vi "Compile Script.vi"(0 "scripts manager in":refnum<class "scripts manager.lvclass">, 11 "error in (no error)":errorcluster) -> (4 "scripts manager out":refnum<class "scripts manager.lvclass">, 15 "error out":errorcluster)   [LabVIEW 2019, in "LSL.lvlib" / "scripts manager.lvclass"]
uses:
  scripts manager.lvclass
  scripts manager.lvclass/scripts manager.ctl
  output terminal/Base/Output Terminal.lvclass
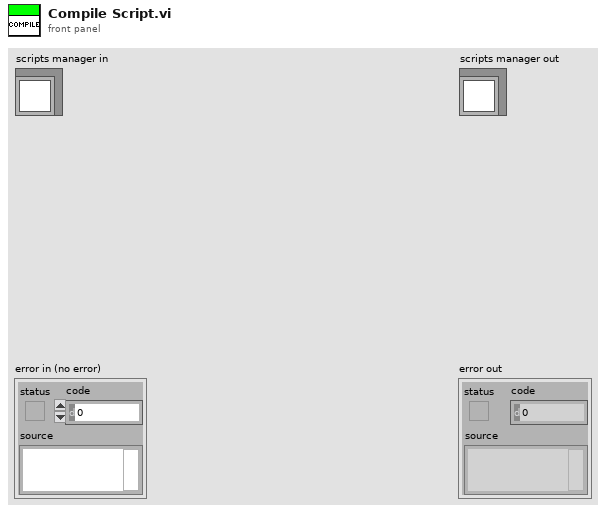
[diagram p1: front panel]
types:
  T1 = typedef "Line Details.ctl" = cluster{"Line#":i64, "Indent#":i64, "Function":string}
  T2 = typedef "Validate_message.ctl" = cluster{"Line Number":i64, "Type":T3, "Message":string}
  T3 = typedef "Validate_MessageStatus.ctl" = enum16{"Message", "Warning", "Error"}
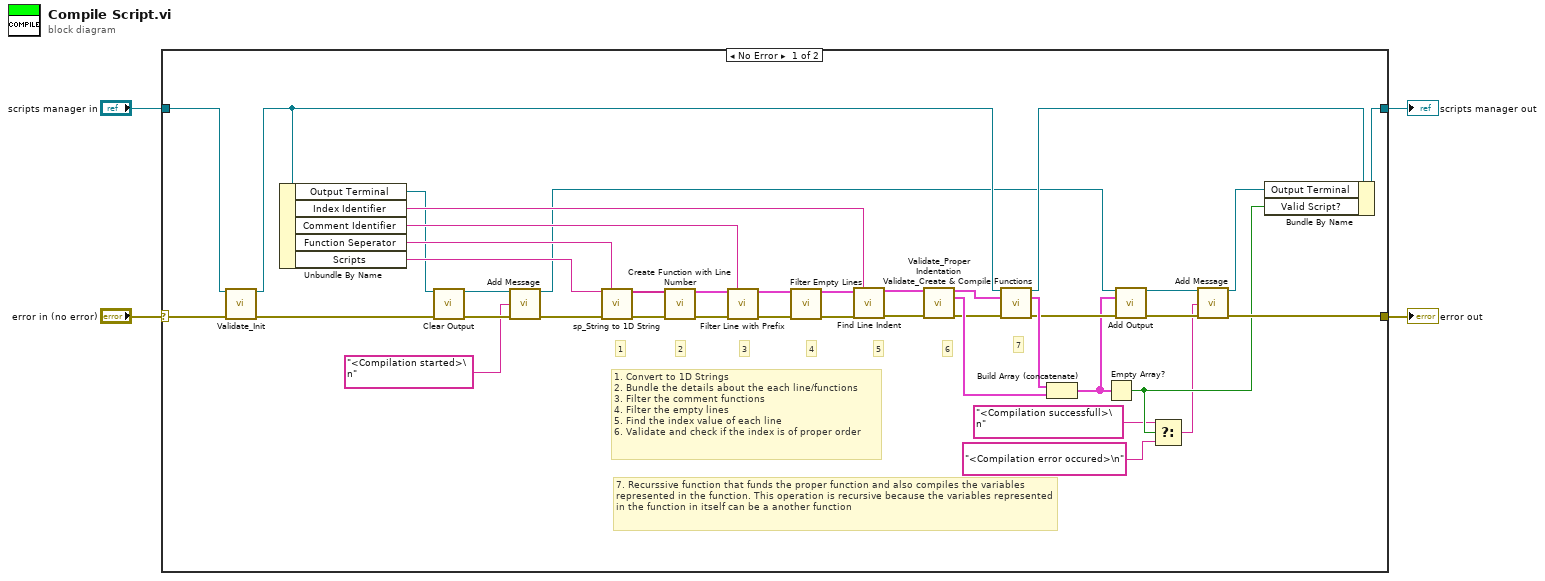
[diagram p0: block diagram]
diagram:
  n1 = case shown="No Error" "error in (no error)" {
    selector: "error in (no error)" -> [w24 w46]
    tunnel: [w10 w46] -> w3
    tunnel: [w31 w45] -> w1
    tunnel: "scripts manager in" -> [w23 w45]
    frame No Error {
      # "7. Recurssive function that funds the proper function and also compiles the variables represented in the function. This operation is recursive because the variables represented in the function in itself can be a another function"
      # "7"
      # "1. Convert to 1D Strings\n2. Bundle the details about the each line/functions\n3. Filter the comment functions\n4. Filter the empty lines\n5. Find the index value of each line\n6. Validate and check if the index is of proper order"
      # "6"
      # "5"
      # "4"
      # "3"
      # "2"
      # "1"
      n2 = call "Validate_Init.vi"("scripts manager in"=w23, "error in (no error)"=w24) -> ("scripts manager out"=w22:refnum<class "scripts manager.lvclass">, "error out"=w18:errorcluster)  [unwired: 12 in]
      n3 = Unbundle By Name(w22) -> ("Output Terminal"=w19:refnum<class "Output Terminal.lvclass">, "Index Identifier"=w33:string, "Comment Identifier"=w38:string, "Function Seperator"=w43:string, "Scripts"=w44:string)
      n4 = call-dynamic "Clear Output.vi"("Output Terminal in"=w19, "error in (no error)"=w18) -> ("Output Terminal out"=w17:refnum<class "Output Terminal.lvclass">, "error out"=w15:errorcluster)  [unwired: 12 in]
      n5 = call-dynamic "Add Message.vi"("Output Terminal in"=w17, "Message"="<Compilation started>\n", "error in (no error)"=w15) -> ("Output Terminal out"=w16:refnum<class "Output Terminal.lvclass">, "error out"=w14:errorcluster)  [unwired: 11 in]
      n6 = call "sp_String to 1D String.vi"("script"=w44, "seperator"=w43, "error in (no error)"=w14) -> ("Script Lines"=w42:string[], "error out"=w41:errorcluster)  [unwired: 11 in]
      n7 = call "Create Function with Line Number.vi"("Script Lines in"=w42, "error in (no error)"=w41) -> ("Functions"=w39:T1[], "error out"=w40:errorcluster)  [unwired: 12 in]
      n8 = call "Filter Line with Prefix.vi"("Functions in"=w39, "Prefix"=w38, "error in (no error)"=w40) -> ("Functions"=w37:T1[], "error out"=w36:errorcluster)  [unwired: 11 in]
      n9 = call "Filter Empty Lines.vi"("Functions in"=w37, "error in (no error)"=w36) -> ("Functions"=w34:T1[], "error out"=w35:errorcluster)  [unwired: 12 in]
      n10 = call "Find Line Indent.vi"("Functions in"=w34, "Indent Identifier"=w33, "error in (no error)"=w35) -> ("Functions"=w29:T1[], "error out"=w32:errorcluster)  [unwired: 11 in]
      n11 = call "Validate_Proper Indentation.vi"("Functions in"=w29, "error in (no error)"=w32) -> ("Functions"=w26:T1[], "Validation message"=w28:T2[], "error out"=w27:errorcluster)  [unwired: 11 in]
      n12 = call "Validate_Create & Compile Functions.vi"("scripts manager in"=w22, "Functions in"=w26, "error in (no error)"=w27) -> ("scripts manager"=w30:refnum<class "scripts manager.lvclass">, "Comiplation message"=w25:T2[], "error out"=w21:errorcluster)  [unwired: 10 in]
      n13 = Build Array (concatenate)(w25, w28) -> (w20:T2[])
      n14 = Empty Array?(array=w20) -> (empty?=w8:bool)
      n15 = call-dynamic "Add Output.vi"("Output Terminal in"=w16, "Comiplation message"=w20, "error in (no error)"=w21) -> ("Output Terminal out"=w12:refnum<class "Output Terminal.lvclass">, "error out"=w11:errorcluster)  [unwired: 11 in]
      n16 = Select(t="<Compilation successfull>\n" ("f"), s=w8, f="<Compilation error occured>\n") -> (s? t:f=w7:string)
      n17 = call-dynamic "Add Message.vi"("Output Terminal in"=w12, "Message"=w7, "error in (no error)"=w11) -> ("Output Terminal out"=w9:refnum<class "Output Terminal.lvclass">, "error out"=w10:errorcluster)  [unwired: 11 in]
      n18 = Bundle By Name(cluster=w30, "Output Terminal"=w9, "Valid Script?"=w8) -> (w31:refnum<class "scripts manager.lvclass">)
    }
    frame Error {
    }
  }
  "error out" <- w3
  "scripts manager out" <- w1
